vi "test_odd_or_even.vi"(1 "input number":i32) -> (0 "even or odd?":T1)   [LabVIEW 2010]
doc: "This VI tests whether an integer is even or odd. It output a corresponding enum value (even/odd)."
uses:
  enumerations/even_odd_enum.ctl
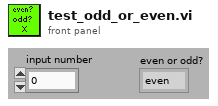
[diagram p1: front panel]
types:
  T1 = typedef "even_odd_enum.ctl" = enum16{"even", "odd"}
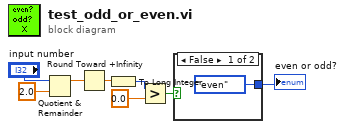
[diagram p0: block diagram]
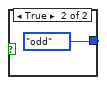
[diagram p2: hidden frame]
diagram:
  n1 = Quotient & Remainder(x="input number", y=2.0) -> (x-y*floor(x/y)=w1:dbl)  [unwired: 1 out]
  n2 = Round Toward +Infinity(x=w1) -> (ceil(x): smallest int >= x=w6:dbl)
  n3 = To Long Integer(number=w6) -> (32bit integer=w4:i32)
  n4 = Greater?(x=w4, y=0.0) -> (0:w3:bool)
  n5 = case shown="False" w3 {
    tunnel: [even_odd_enum."even" ("even or odd?") even_odd_enum."odd" ("even or odd?")] -> w2
    frame False {
    }
    frame True {
    }
  }
  "even or odd?" <- w2
